vi "TangoConnect.vi"() -> ()   [LabVIEW 2018]
panel:
  out "plLSID out":i32
  out "success":bool
  out "error out":errorcluster
  in  "show Protocol":bool
  out "Baud":dbl
  in  "Tango Com":refnum<visa-resource-name>
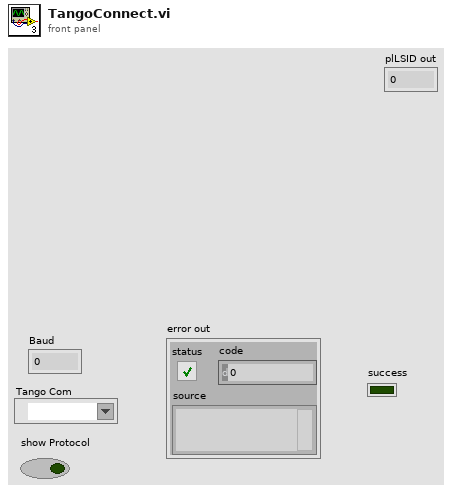
[diagram p1: front panel]
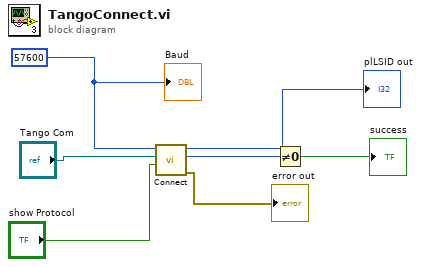
[diagram p0: block diagram]
diagram:
  w7 = 57600 ("lABaudRate")
  n1 = call "Connect.vi"("ShProt?"="show Protocol", "pcAComName"="Tango Com", "lABaudRate"=w7) -> ("error out"=→"error out":errorcluster, "function return"=w3:i32, "plLSID out"=→"plLSID out":i32)  [unwired: 5 in]
  n2 = Not Equal To 0?(x=w3) -> (x != 0?=→"success":bool)
  "Baud" <- w7
